vi "NavX Global.vi"() -> ()   [LabVIEW 2016]
panel:
  out "NavX Displacement":T1
  in  "Robot Angle":dbl
  out "NaxX Gyro":T2
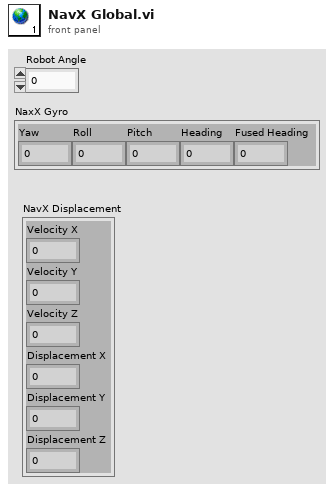
[diagram p1: front panel]
types:
  T1 = cluster{"Velocity X":dbl, "Velocity Y":dbl, "Velocity Z":dbl, "Displacement X":dbl, "Displacement Y":dbl, "Displacement Z":dbl}
  T2 = cluster{"Yaw":dbl, "Roll":dbl, "Pitch":dbl, "Heading":dbl, "Fused Heading":dbl}
diagram:
